vi "add keypair from file.vi"(8 "error in":errorcluster, 9 "key":path, 10 "cert":path, 11 "lvlibretls server listener in":refnum<class "lvlibretls server listener.lvclass">) -> (0 "error out":errorcluster, 3 "lvlibretls server listener out":refnum<class "lvlibretls server listener.lvclass">)   [LabVIEW 2016, in "lvlibretls server listener.lvclass"]
uses:
  lvlibretls server listener.lvclass
  C:/Users/IEUser/Desktop/tlssimple/libretls/context parent/lvlibretls configurable context.lvclass
  context parent/lvlibretls configurable context.lvclass/lvlibretls configurable context.ctl
  context parent/lvlibretls configurable context.lvclass
  lv tls dll.lvlib
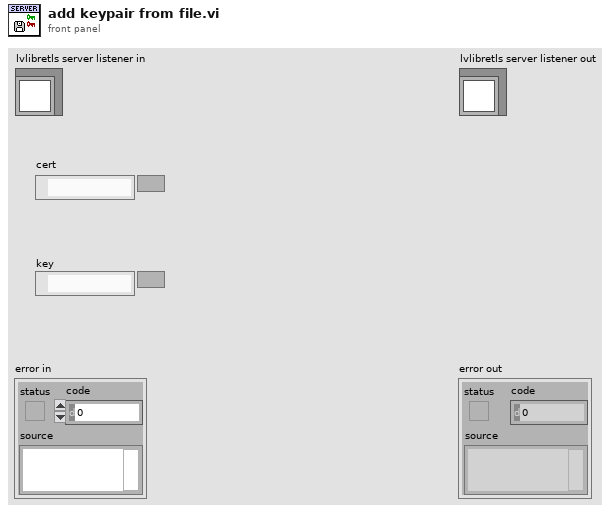
[diagram p1: front panel]
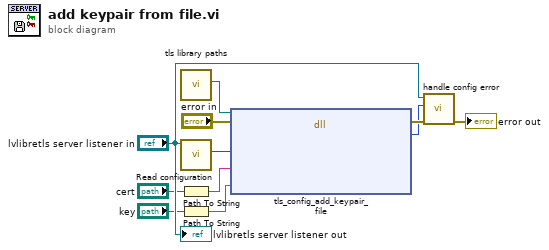
[diagram p0: block diagram]
diagram:
  n1 = call "tls library paths.vi"() -> ("libtls"=w10:path)  [unwired: 8 in, 3 out]
  n2 = call "Read configuration.vi"("lvlibretls configurable context in"="lvlibretls server listener in") -> ("configuration"=w9:u64)  [unwired: 10 in]
  n3 = Path To String(path="cert") -> (string=w1:string)
  n4 = Path To String(path="key") -> (string=w2:string)
  n5 = dll-call lib="C:/Users/IEUser/Desktop/tlssimple/libtls-15.dll" fn="tls_config_add_keypair_file"(path in=w10, error in="error in", "config"=w9, "certfile"=w1, "keyfile"=w2) -> (error out=w8:errorcluster, "return"=w5:i32)  [unwired: 4 in, 1 out]
  n6 = call "handle config error.vi"("error in"=w8, "return"=w5, "lvlibretls configurable context in"="lvlibretls server listener in") -> ("error out"=→"error out":errorcluster)  [unwired: 8 in]
  "lvlibretls server listener out" <- "lvlibretls server listener in"
